vi "Framework_Initialize.vi"(8 "error in (no error)":errorcluster, 11 "AB_InteropAssembly in":refnum<class "AB_InteropAssembly.lvclass">) -> (0 "error out":errorcluster, 1 "helpTopics":string[](array[string]), 2 "pageTitles":string[](array[string]), 3 "AB_InteropAssembly out":refnum<class "AB_InteropAssembly.lvclass">, 4 "helpFile":string, 5 "pages":path[](array[path]))   [LabVIEW 2020, in "AB_InteropAssembly.lvclass"]
uses:
  <vilib>/AppBuilder/AB_Classes/InteropAssembly/AB_InteropAssembly.lvclass
panel:
  in  "pageTitles_Assembly":string[](array[string])=["Information", "Source Files", "Destinations", "Source File Settings", "Advanced", "Additional Exclusions", "Version Information", "Windows Security", "Run-Time Languages", "Pre/Post Build Actions", "Preview"]
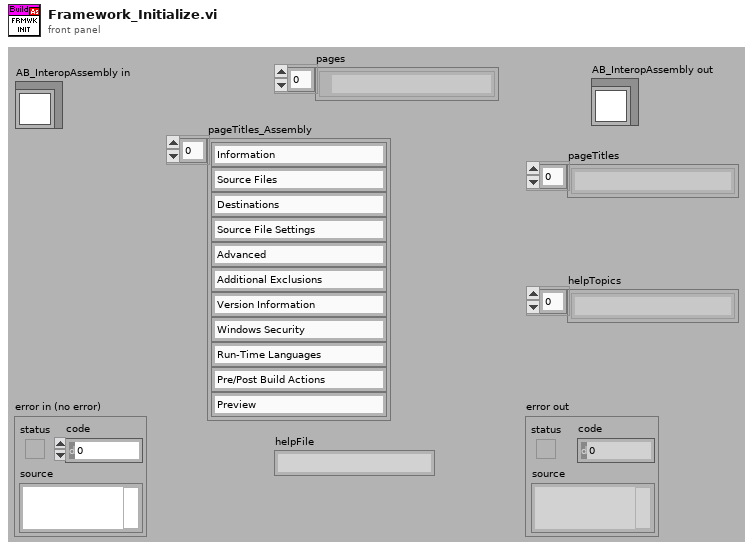
[diagram p1: front panel]
types:
  T1 = enum32{"invalid OS target", "Mac OS", "Windows 3.1", "Windows 95/NT", "Solaris 1", "Solaris 2", "HP-UX", "PowerMAX", "Linux", "Irix", "Rhapsody", "BeOS", "AIX", "OSF1", "VxWorks", "PharLap", "Carbon", "RTX", "Windows x64", "Linux x64", "Mac OS X x64"}
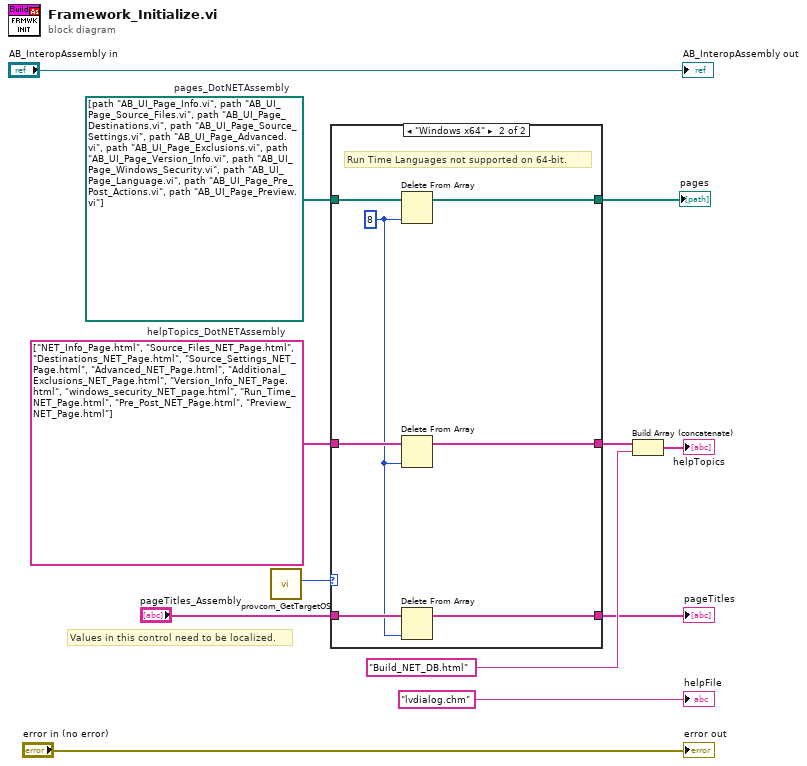
[diagram p0: block diagram]
diagram:
  w6 = string[] ["NET_Info_Page.html", "Source_Files_NET_Page.html", "Destinations_NET_Page.html", "Source_Settings_NET_Page.html", "Advanced_NET_Page.html", "Additional_Exclusions_NET_Page.html", "Version_Info_NET_Page.html", "windows_security_NET_page.html", "Run_Time_NET_Page.html", "Pre_Post_NET_Page.html", "Preview_NET_Page.html"]  # helpTopics_DotNETAssembly
  w5 = path[] [path "AB_UI_Page_Info.vi", path "AB_UI_Page_Source_Files.vi", path "AB_UI_Page_Destinations.vi", path "AB_UI_Page_Source_Settings.vi", path "AB_UI_Page_Advanced.vi", path "AB_UI_Page_Exclusions.vi", path "AB_UI_Page_Version_Info.vi", path "AB_UI_Page_Windows_Security.vi", path "AB_UI_Page_Language.vi", path "AB_UI_Page_Pre_Post_Actions.vi", path "AB_UI_Page_Preview.vi"]  # pages_DotNETAssembly
  # "8"
  # "Values in this control need to be localized."
  n1 = call <resource>:"provcom_GetTargetOS.vi"() -> ("App.TargetOS"=w4:T1)  [unwired: 11 out]
  n2 = case shown="\"Windows x64\"" w4 {
    tunnel: "pageTitles_Assembly" -> [w13 w18]
    tunnel: w6 -> [w14 w20]
    tunnel: w5 -> [w15 w22]
    tunnel: [w15 w21] -> w3
    tunnel: [w14 w19] -> w2
    tunnel: [w13 w17] -> w1
    frame Default {
    }
    frame "Windows x64" {
      w16 = 8 ("length")
      # "Run Time Languages not supported on 64-bit."
      n3 = Delete From Array(array=w22, index=w16) -> (array with subset deleted=w21:path[])  [unwired: 1 in, 1 out]
      n4 = Delete From Array(array=w20, index=w16) -> (array with subset deleted=w19:string[])  [unwired: 1 in, 1 out]
      n5 = Delete From Array(array=w18, index=w16) -> (array with subset deleted=w17:string[])  [unwired: 1 in, 1 out]
    }
  }
  "pages" <- w3
  "pageTitles" <- w1
  n6 = Build Array (concatenate)(w2, "Build_NET_DB.html" ("HTML filename")) -> (→"helpTopics":string[])
  "error out" <- "error in (no error)"
  "helpFile" <- "lvdialog.chm" ("CHM or HLP filename (lvdialog.chm)")
  "AB_InteropAssembly out" <- "AB_InteropAssembly in"
